vi "BRig_RT_comm_NetStream_testConnect.vi"() -> ()   [LabVIEW 2014]
panel:
  out "error out":errorcluster
  in  "stop":bool
  out "Sending":bool
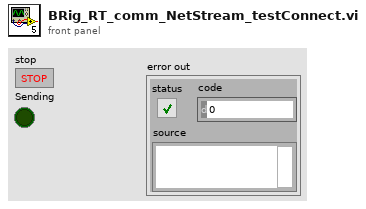
[diagram p1: front panel]
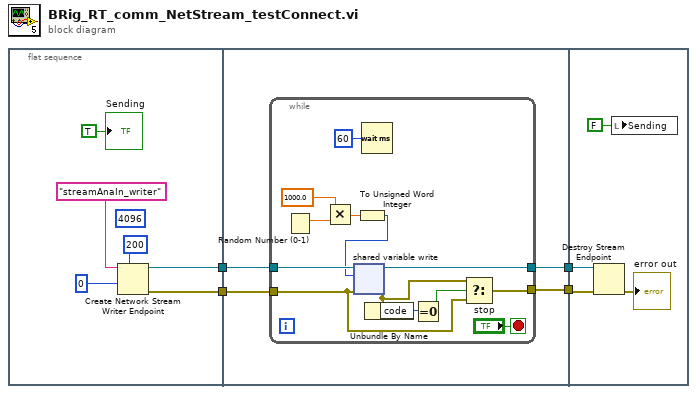
[diagram p0: block diagram]
diagram:
  n1 = flat-sequence {
    tunnel: [w6] -> w4
    tunnel: [w5] -> w3
    tunnel: w4 -> [w14]
    tunnel: w3 -> [w13]
    tunnel: [w12] -> w2
    tunnel: [w11] -> w1
    tunnel: w2 -> [w30]
    tunnel: w1 -> [w29]
    frame #0 {
      (unwired) 4096 ("reader buffer size")
      n2 = Create Network Stream Writer Endpoint(7:200 ("reader buffer size"), 9:u16 0 ("element"), 11:"streamAnaIn_writer" ("reader name")) -> (0:w5:errorcluster, 3:w6:refnum<k21>)  [unwired: 4 in]
      "Sending" <- TRUE ("Sending")
    }
    frame #1 {
      n3 = while {
        tunnel: w14 -> [w27]
        tunnel: w13 -> [w18]
        tunnel: [w21] -> w12
        tunnel: [w16] -> w11
        stop <- "stop" stop-if-true
        n4 = Random Number (0-1)() -> (number: 0 to 1=w26:dbl)
        n5 = Multiply(x=1000.0, y=w26) -> (x*y=w24:dbl)
        n6 = To Unsigned Word Integer(number=w24) -> (unsigned 16bit integer=w23:u16)
        n7 = shared-variable-write(w27, w18, w23) -> (w21:refnum<k21>, w17:errorcluster)  [unwired: 1 in, 1 out]
        n8 = Wait (ms)(milliseconds to wait=u32 60) -> ()  [unwired: 1 out]
        n9 = Unbundle By Name(w17) -> ("code"=w22:i32)
        n10 = Equal To 0?(x=w22) -> (x = 0?=w19:bool)
        n11 = Select(t=w17, s=w19, f=w18) -> (s? t:f=w16:errorcluster)
      }
    }
    frame #2 {
      n12 = Destroy Stream Endpoint(8:w29, 11:w30) -> (0:→"error out":errorcluster)
      n13 = local write "Sending"(FALSE ("Sending")) -> ()
    }
  }
